vi "Thread@ErrorRetry__Parameter.vi"(1 "ParamterIn":string) -> (0 "ParamterOut":string)   [LabVIEW 2019]
panel:
  out "IO List":string[](array[string])
  in  "Offset":string(combo)
  in  "Logic":string(combo)
  in  "Confirm":bool
  # "Thread@ErrorRetry ($Logic,$ReturnOffset)"
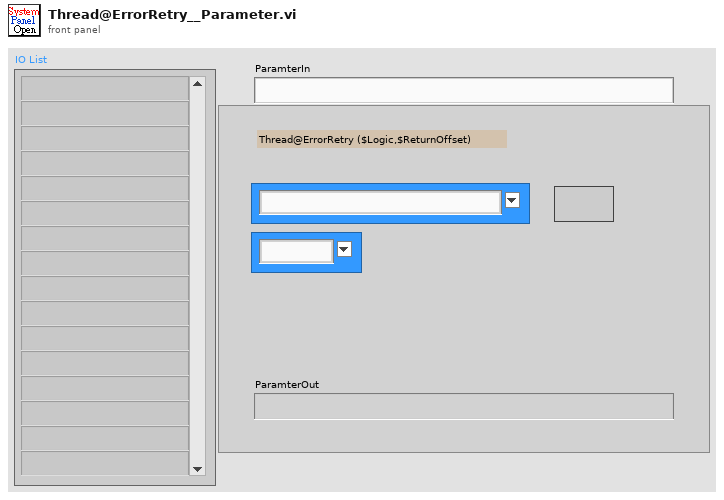
[diagram p1: front panel]
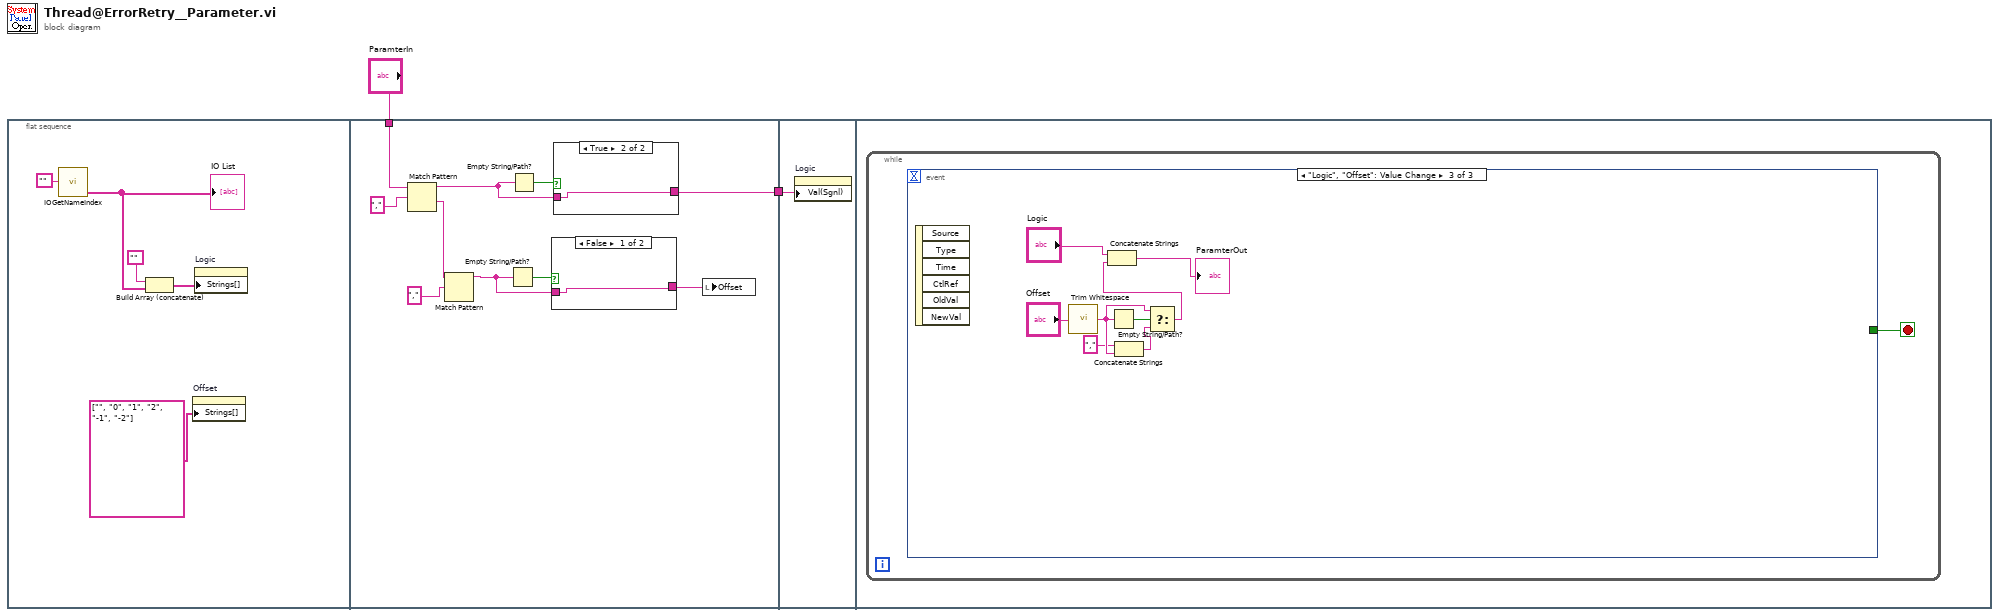
[diagram p0: block diagram]
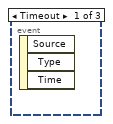
[diagram p4: hidden frame]
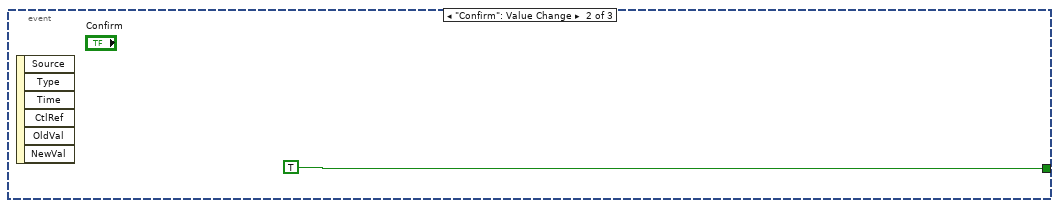
[diagram p5: hidden frame]
diagram:
  n1 = flat-sequence {
    tunnel: "ParamterIn" -> [w16]
    tunnel: [w12] -> w1
    tunnel: w1 -> [w22]
    frame #0 {
      n2 = call "IOGetNameIndex.vi"("PortName"="") -> ("PortNameList Out"=w6:string[])  [unwired: 3 in, 1 out]
      "IO List" <- w6
      n3 = Build Array (concatenate)("", w6) -> (w4:string[])
      n4 = property on="Offset" class="CmbBox"("Strings[]"=string[] ["", "0", "1", "2", "-1", "-2"] ("Strings []")) -> ()  [unwired: 2 in, 2 out]
      n5 = property on="Logic" class="CmbBox"("Strings[]"=w4) -> ()  [unwired: 2 in, 2 out]
    }
    frame #1 {
      n6 = Match Pattern(string=w16, regular expression=",") -> (before substring=w14:string, after substring=w9:string)  [unwired: 1 in, 2 out]
      n7 = Match Pattern(string=w9, regular expression=",") -> (before substring=w8:string)  [unwired: 1 in, 3 out]
      n8 = Empty String/Path?(string/path=w8) -> (empty?=w13:bool)
      n9 = Empty String/Path?(string/path=w14) -> (empty?=w17:bool)
      n10 = case shown="False" w13 {
        tunnel: w8 -> [w18 w19]
        tunnel: [w18 w19] -> w11
        frame False {
        }
        frame True {
        }
      }
      n11 = case shown="True" w17 {
        tunnel: w14 -> [w20 w21]
        tunnel: [w20 w21] -> w12
        frame False {
        }
        frame True {
        }
      }
      n12 = local write "Offset"(w11) -> ()
    }
    frame #2 {
      n13 = property on="Logic" class="CmbBox"("Val(Sgnl)"=w22) -> ()  [unwired: 2 in, 2 out]
    }
    frame #3 {
      n14 = while {
        stop <- w23 stop-if-true
        n15 = event shown="[2] \"Logic\", \"Offset\": Value Change" {
          selector: _ -> [_ _ _]
          dyn-events: _ -> [_ _ _]
          timeout: _ -> [_ _ _]
          tunnel: [_ TRUE _] -> w23
          event Timeout {
            n16 = event-data() -> ()  [unwired: 1 in, 3 out]
          }
          event "Confirm": Value Change {
            n17 = event-data() -> ()  [unwired: 1 in, 6 out]
          }
          event "Logic", "Offset": Value Change {
            n18 = event-data() -> ()  [unwired: 1 in, 6 out]
            n19 = call <vilib>:"Trim Whitespace.vi"("string"="Offset") -> ("trimmed string"=w27:string)  [unwired: 1 in]
            n20 = Empty String/Path?(string/path=w27) -> (empty?=w29:bool)
            n21 = Concatenate Strings("," ("string"), w27) -> (w28:string)
            n22 = Select(t=w27, s=w29, f=w28) -> (s? t:f=w25:string)
            n23 = Concatenate Strings("Logic", w25) -> (→"ParamterOut":string)
          }
        }
      }
    }
  }
